vi "Create.vi"(8 "error in (no error)":errorcluster, 11 "msg":refnum<k7>) -> (0 "error out":errorcluster, 2 "Code":T1, 3 "UIMessage out":refnum<class "UIMessage.lvclass">)   [LabVIEW 2020, in "TSS.lvlib" / "UIMessage.lvclass"]
uses:
  UIMessage.lvclass
  Data Types/UIMsg.ctl
  UIMessage.lvclass/UIMessage.ctl
  TSS.lvlib
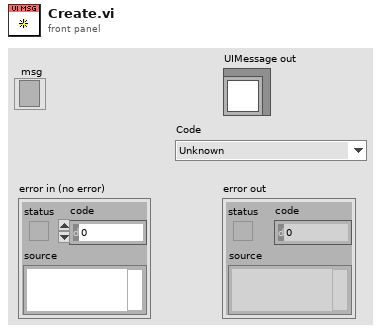
[diagram p1: front panel]
types:
  T1 = typedef "TSS.lvlib/UIMsg.ctl" = enum16{"Unknown", "BreakOnUserRequest", "BreakOnBreakpoint", "BreakOnRunTimeError", "Trace", "TerminatingExecution", "AbortingExecution", "KillingExecutionThreads", "EndExecution", "ShutDownComplete", "StartExecution", "ProgressPercent", "ProgressText", "StartInteractiveExecution", "EndInteractiveExecution", "TerminatingInteractiveExecution", "TerminationCancelled", "ResumeFromBreak", "StartFileExecution", "EndFileExecution", "ShutDownCancelled", "LocalizationSettingChanged", "OpenWindows", "TileWindows", "CascadeWindows", "ReportChanged", "CloseWindows", "RefreshWindows", "ClientFileChanged", "DisplayReport", "ModelState_Initializing", "ModelState_Waiting", "ModelState_Identified", "ModelState_BeginTesting", "ModelState_TestingComplete", "ModelState_PostProcessingComplete", "ModelState_EnabledStateSet", "ReportLocationChanged", "GotoLocation", "PushUndoItem", "OutputMessages", "TypePaletteFileListChanged", "NonTerminatingThreadsArePreventingTermination", "ModelState_PostProcessing", "ReportCollectionChanged", "RuntimeError"}
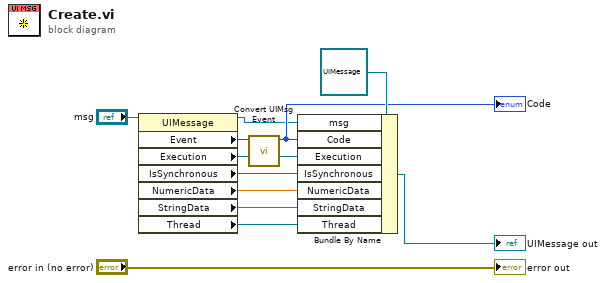
[diagram p0: block diagram]
diagram:
  n1 = property class="UIMessage"(reference="msg") -> (reference out=w1:refnum<k7>, "Event"=w9:i32, "Execution"=w6:refnum<k7>, "IsSynchronous"=w2:bool, "NumericData"=w3:dbl, "StringData"=w4:string, "Thread"=w5:refnum<k7>)  [unwired: 1 in, 1 out]
  n2 = call "Convert UIMsg Event.vi"("UIMsg Event"=w9) -> ("UIMsg"=w7:T1)  [unwired: 9 in, 1 out]
  "Code" <- w7
  n3 = Bundle By Name(cluster=refnum<class "UIMessage.lvclass"> refnum ("UIMessage in"), "msg"=w1, "Code"=w7, "Execution"=w6, "IsSynchronous"=w2, "NumericData"=w3, "StringData"=w4, "Thread"=w5) -> (→"UIMessage out":refnum<class "UIMessage.lvclass">)
  "error out" <- "error in (no error)"
